vi "Set Dut Selectors.vi"(8 "error in":errorcluster, 9 "SWD Sel Task":refnum<k21>, 10 "Dut Selector":bool, 11 "RF Switch Sel Task":refnum<k21>) -> (0 "error out":errorcluster)   [LabVIEW 2018]
uses:
  <vilib>/DAQmx/write.llb/DAQmx Write (Digital Bool 1Line 1Point).vi
  <vilib>/DAQmx/write.llb/DAQmx Write (Digital 1D Bool 1Chan 1Samp).vi
  <vilib>/DAQmx/miscellaneous.llb/DAQmx Fill In Error Info.vi
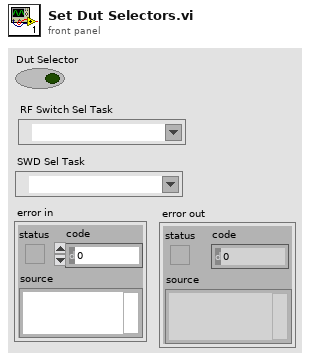
[diagram p1: front panel]
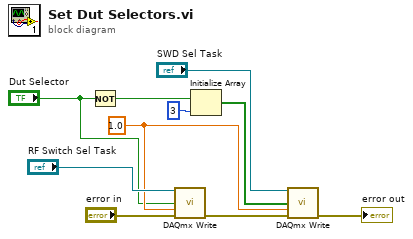
[diagram p0: block diagram]
diagram:
  w4 = 1.0 ("timeout")
  n1 = Not(x="Dut Selector") -> (.not. x?=w1:bool)
  n2 = call-poly <vilib>:"DAQmx Write.vi"("task/channels in"="RF Switch Sel Task", "data"="Dut Selector", "timeout"=w4, "error in"="error in") -> ("error out"=w6:errorcluster)  [unwired: 9 in, 2 out]
  n3 = Initialize Array(w1, 3 ("dimension size")) -> (w3:bool[])
  n4 = call-poly <vilib>:"DAQmx Write.vi"("task/channels in"="SWD Sel Task", "data"=w3, "timeout"=w4, "error in"=w6) -> ("error out"=→"error out":errorcluster)  [unwired: 9 in, 2 out]
